vi "Insert Version.vi"(8 "error in (no error)":errorcluster, 9 "index":i32, 10 "Build Type":T1=enum."Build", 11 "Builder in":refnum<class "Builder.lvclass">) -> (0 "error out":errorcluster, 3 "Builder out":refnum<class "Builder.lvclass">)   [LabVIEW 2021, in "App-Builder Library.lvlib" / "Builder.lvclass"]
uses:
  Builder.lvclass
  Build Type.ctl
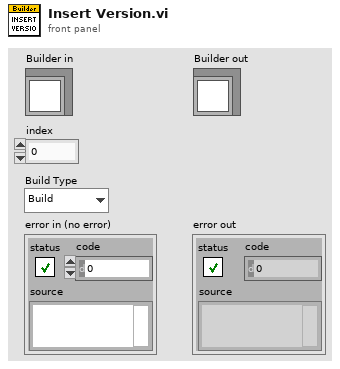
[diagram p1: front panel]
types:
  T1 = typedef "App-Builder Library.lvlib/Builder.lvclass/Build Type.ctl" = enum16{"Major", "Minor", "Fix", "Build"}
  T2 = typedef "NI_App_Builder_API.lvlib/Build Specification Version.ctl" = cluster{"Major":u16, "Minor":u16, "Fix":u16, "Build":u16}
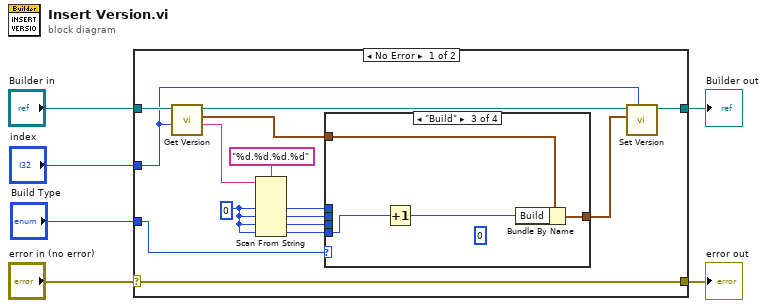
[diagram p0: block diagram]
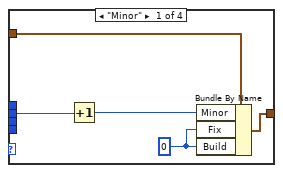
[diagram p2: hidden frame]
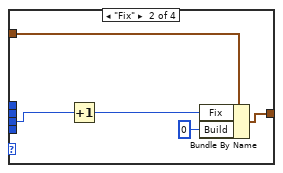
[diagram p3: hidden frame]
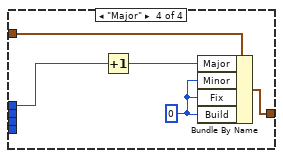
[diagram p4: hidden frame]
diagram:
  n1 = case shown="No Error" "error in (no error)" {
    selector: "error in (no error)" -> [w21 w42]
    tunnel: [w21 w42] -> w5
    tunnel: [w20 w41] -> w3
    tunnel: "Builder in" -> [w18 w41]
    tunnel: "index" -> [w7 _]
    tunnel: "Build Type" -> [w16 _]
    frame No Error {
      w8 = u16 0 ("Build")
      n2 = call-dynamic "Get Version.vi"("index"=w7, "Builder in"=w18) -> ("Build Version (String)"=w10:string, "Build Version"=w9:T2, "Builder out"=w17:refnum<class "Builder.lvclass">)  [unwired: 6 in, 1 out]
      n3 = Scan From String(format string="%d.%d.%d.%d", input string=w10, default 1=w8, default 2=w8, default 3=w8, default 4=w8) -> (output 1=w14:u16, output 2=w13:u16, output 3=w12:u16, output 4=w11:u16)  [unwired: 2 in, 3 out]
      n4 = case shown="\"Build\"" w16 {
        tunnel: [w26 w31 w35 w40] -> w19
        tunnel: w14 -> [_ _ _ w37]
        tunnel: w13 -> [w24 _ _ _]
        tunnel: w12 -> [_ w28 _ _]
        tunnel: w11 -> [_ _ w33 _]
        tunnel: w9 -> [w25 w30 w34 w39]
        frame "Minor" {
          w22 = u16 0 ("Build")
          n5 = Increment(x=w24) -> (x+1=w23:u16)
          n6 = Bundle By Name(cluster=w25, "Minor"=w23, "Fix"=w22, "Build"=w22) -> (w26:T2)
        }
        frame "Fix" {
          n7 = Increment(x=w28) -> (x+1=w29:u16)
          n8 = Bundle By Name(cluster=w30, "Fix"=w29, "Build"=u16 0) -> (w31:T2)
        }
        frame "Build" {
          (unwired) u16 0 ("x+1")
          n9 = Increment(x=w33) -> (x+1=w32:u16)
          n10 = Bundle By Name(cluster=w34, "Build"=w32) -> (w35:T2)
        }
        frame "Major" {
          w36 = u16 0 ("Minor")
          n11 = Increment(x=w37) -> (x+1=w38:u16)
          n12 = Bundle By Name(cluster=w39, "Major"=w38, "Minor"=w36, "Fix"=w36, "Build"=w36) -> (w40:T2)
        }
      }
      n13 = call "Set Version.vi"("Index"=w7, "Build Version"=w19, "Builder in"=w17) -> ("Builder out"=w20:refnum<class "Builder.lvclass">)  [unwired: 7 in, 1 out]
    }
    frame Error {
    }
  }
  "error out" <- w5
  "Builder out" <- w3
